vi "create_static_waveform.vi"(0 "Waveform Parameters":T1={"Constant"=1.0, "Nickname"="", "Conversion"=enum."B Field Grad (G/cm)"}, 1 "Sample rate":dbl, 2 "Time":dbl) -> (3 "Samples to Write":dbl, 4 "dt":dbl, 6 "output waveform":waveform(dbl)(graph))   [LabVIEW 2016]
uses:
  Controls/6713/6713_static_waveform_item.ctl
  6733_Red_MOT/Neutral_voltage_conversion_control.ctl
panel:
  out "Numeric":i32
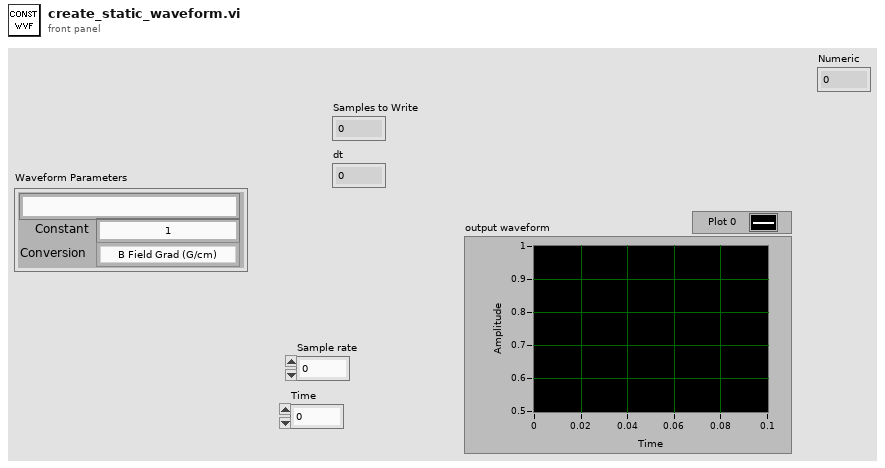
[diagram p1: front panel]
types:
  T1 = typedef "6713_static_waveform_item.ctl" = cluster{"Constant":dbl, "Nickname":string, "Conversion":T2}
  T2 = typedef "Neutral_voltage_conversion_control.ctl" = enum16{"Volts", "B Field Grad (G/cm)", "Red Boson Cntr Freq (MHz)", "Red Boson Dither Amp (kHz)", "Red Boson Power (mW)", "Red 87 Trap Cntr Freq (MHz)", "Red 87 Trap Dither Amp (kHz)", "Red 87 Trap Power (mW)", "Red 87 Stir Cntr Freq (MHz)", "Red 87 Stir Dither Amp (kHz)", "Red 87 Stir Power (mW)", "ODT Sheet Trap Power (W)", "ODT Loading Trap Power (W)"}
  T3 = cluster{"Waveform Parameters":T1, "Time":dbl, "Sample rate":dbl}
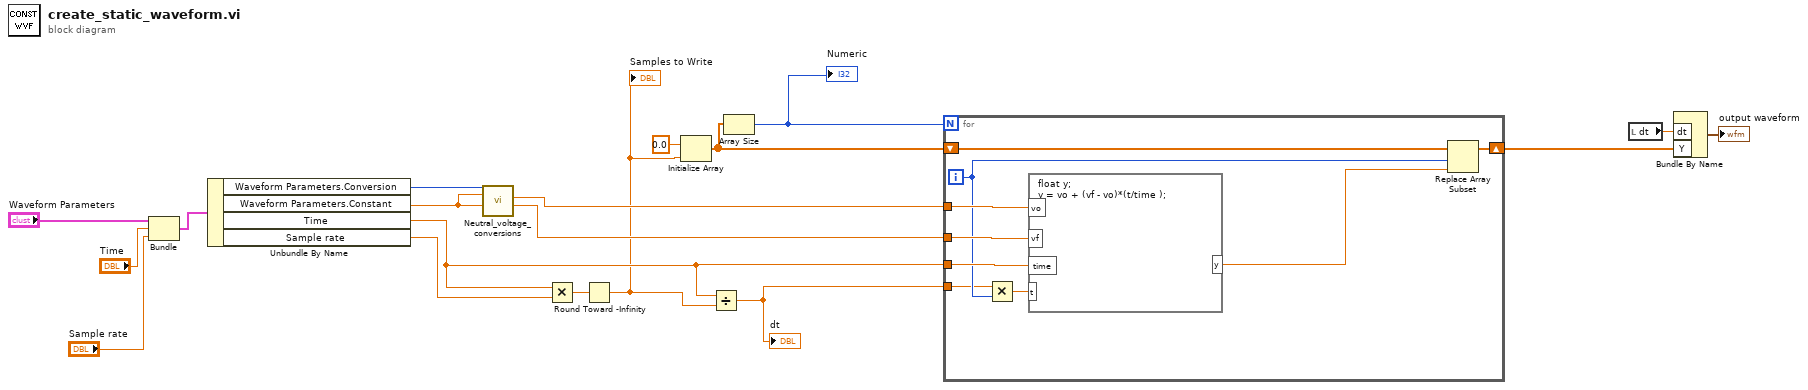
[diagram p0: block diagram]
diagram:
  n1 = Bundle("Waveform Parameters"="Waveform Parameters", "Time"="Time", "Sample rate"="Sample rate") -> (w8:T3)  [unwired: 1 in]
  n2 = Unbundle By Name(w8) -> ("Waveform Parameters.Conversion"=w7:T2, "Waveform Parameters.Constant"=w2:dbl, "Time"=w14:dbl, "Sample rate"=w4:dbl)
  n3 = call "Neutral_voltage_conversions.vi"("Final Value"=w2, "Initial value"=w2, "Conversion"=w7) -> ("Final Voltage"=w5:dbl, "Initial voltage"=w6:dbl)  [unwired: 7 in]
  n4 = Multiply(x=w14, y=w4) -> (x*y=w12:dbl)
  n5 = Round Toward -Infinity(1:w12) -> (0:w3:dbl)
  "Samples to Write" <- w3
  n6 = Initialize Array(0.0 ("element"), w3) -> (w15:dbl[])
  n7 = Divide(x=w14, y=w3) -> (x/y=w1:dbl)
  "dt" <- w1
  n8 = Array Size(array=w15) -> (size(s)=w13:i32)
  "Numeric" <- w13
  n9 = for {
    N: w13 -> [_]
    shift-right: [w27] -> w18
    shift-left: w15 -> [w28]
    tunnel: w6 -> [w26]
    tunnel: w5 -> [w25]
    tunnel: w14 -> [w24]
    tunnel: w1 -> [w21]
    i -> [w22]
    n10 = Multiply(x=w21, y=w22) -> (x*y=w23:dbl)
    n11 = formula code="float y;\ny = vo + (vf - vo)*(t/time );"("vo"=w26, "vf"=w25, "time"=w24, "t"=w23) -> ("y"=w20:dbl)
    n12 = Replace Array Subset(array=w28, new element=w20, index=w22) -> (w27:dbl[])
  }
  n13 = local read "dt"() -> (w17:dbl)
  n14 = Bundle By Name("dt"=w17, "Y"=w18) -> (→"output waveform":waveform(dbl))  [unwired: 1 in]
